vi "Open Safety Relay.vi"(8 "error in (no error)":errorcluster, 11 "Test Stand in":refnum<class "Cryo Sep Test Stand.lvclass">) -> (0 "error out":errorcluster, 3 "Test Stand out":refnum<class "Cryo Sep Test Stand.lvclass">)   [LabVIEW 2019, in "Test Stands.lvlib" / "Cryo Sep Test Stand.lvclass"]
uses:
  Cryo Sep Test Stand.lvclass
  Cryo Sep Test Stand.lvclass/Cryo Sep Test Stand.ctl
  <vilib>/DAQmx/write.llb/DAQmx Write (Analog DBL 1Chan 1Samp).vi
  <vilib>/DAQmx/miscellaneous.llb/DAQmx Fill In Error Info.vi
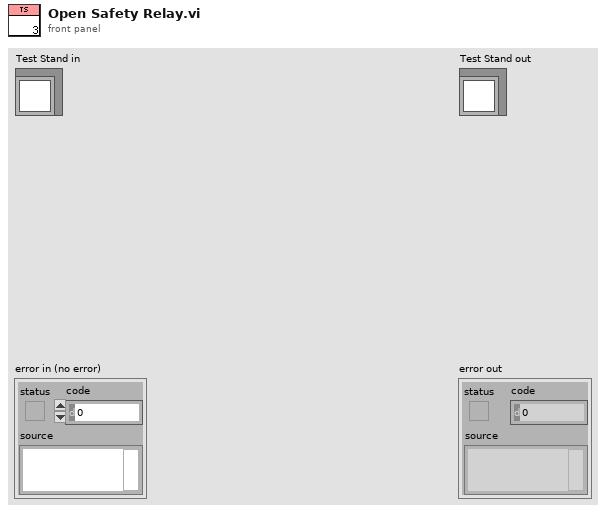
[diagram p1: front panel]
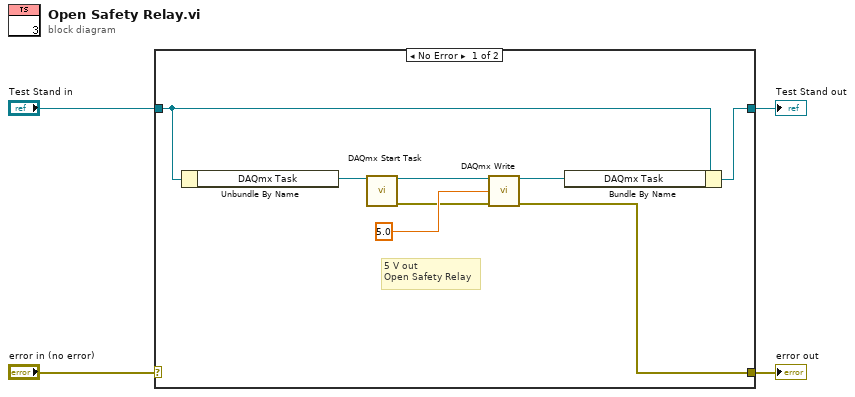
[diagram p0: block diagram]
diagram:
  n1 = case shown="No Error" "error in (no error)" {
    selector: "error in (no error)" -> [_ w14]
    tunnel: [w5 w14] -> w3
    tunnel: [w6 w13] -> w1
    tunnel: "Test Stand in" -> [w8 w13]
    frame No Error {
      # "5 V out\nOpen Safety Relay"
      n2 = Unbundle By Name(w8) -> ("DAQmx Task"=w12:refnum<k21>)
      n3 = call <vilib>:"DAQmx Start Task.vi"("task/channels in"=w12) -> ("task out"=w11:refnum<k21>, "error out"=w9:errorcluster)  [unwired: 13 in]
      n4 = call-poly <vilib>:"DAQmx Write.vi"("task/channels in"=w11, "data"=5.0, "error in"=w9) -> ("task out"=w7:refnum<k21>, "error out"=w5:errorcluster)  [unwired: 10 in, 1 out]
      n5 = Bundle By Name(cluster=w8, "DAQmx Task"=w7) -> (w6:refnum<class "Cryo Sep Test Stand.lvclass">)
    }
    frame Error {
    }
  }
  "error out" <- w3
  "Test Stand out" <- w1
